vi "ExeCmd_async.vi"(4 "HighPrio":bool, 6 "CmdVIRef":refnum<vi>, 8 "ErrorIn":errorcluster, 9 "NameOfVi2Call(optional)":string, 10 "CmdData":variant, 11 "YActorIn":refnum<class "YActor.lvclass">) -> (0 "ErrorOut":errorcluster)   [LabVIEW 2021, in "YActor.lvclass"]
uses:
  YActor.lvclass
  YActor.lvclass/YActor.ctl
  private/CmdCtrl.ctl
  AsyncErrorHandling.ctl
  private/CallMode.ctl
  private/VINameProperty.vi
  InlineReferencePool.vi
panel:
  # "Do not use this VI in a loop where different Cmd VI references are routed.\nThis will cause the execution of the first called command VI only"
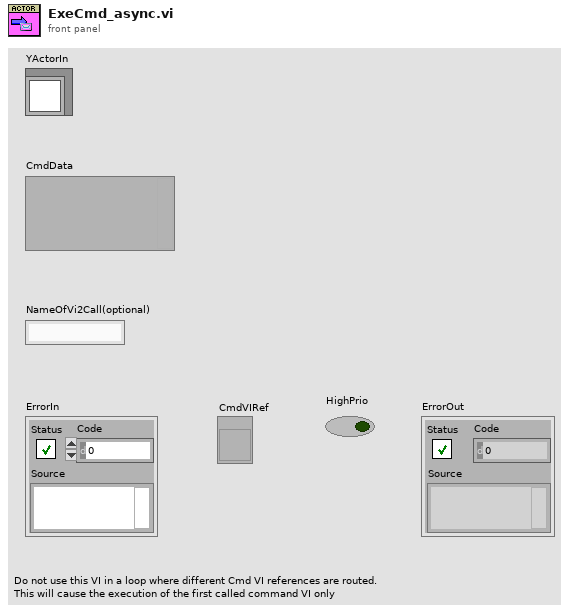
[diagram p1: front panel]
types:
  T1 = typedef "YActor.lvclass/CallMode.ctl" = enum16{"Standard", "Call&Collect"}
  T2 = typedef "YActor.lvclass/CmdCtrl.ctl" = cluster{"CmdData":variant, "CommandVI":string, "ReplyQ":i64, "Error":errorcluster, "Msg#":u32, "AsyncErrorHandling":T3, "CallMode":T1, "Source":string}
  T3 = typedef "YActor.lvclass/AsyncErrorHandling.ctl" = enum16{"Return after executing sync command", "Return before executing sync command", "Don't return error"}
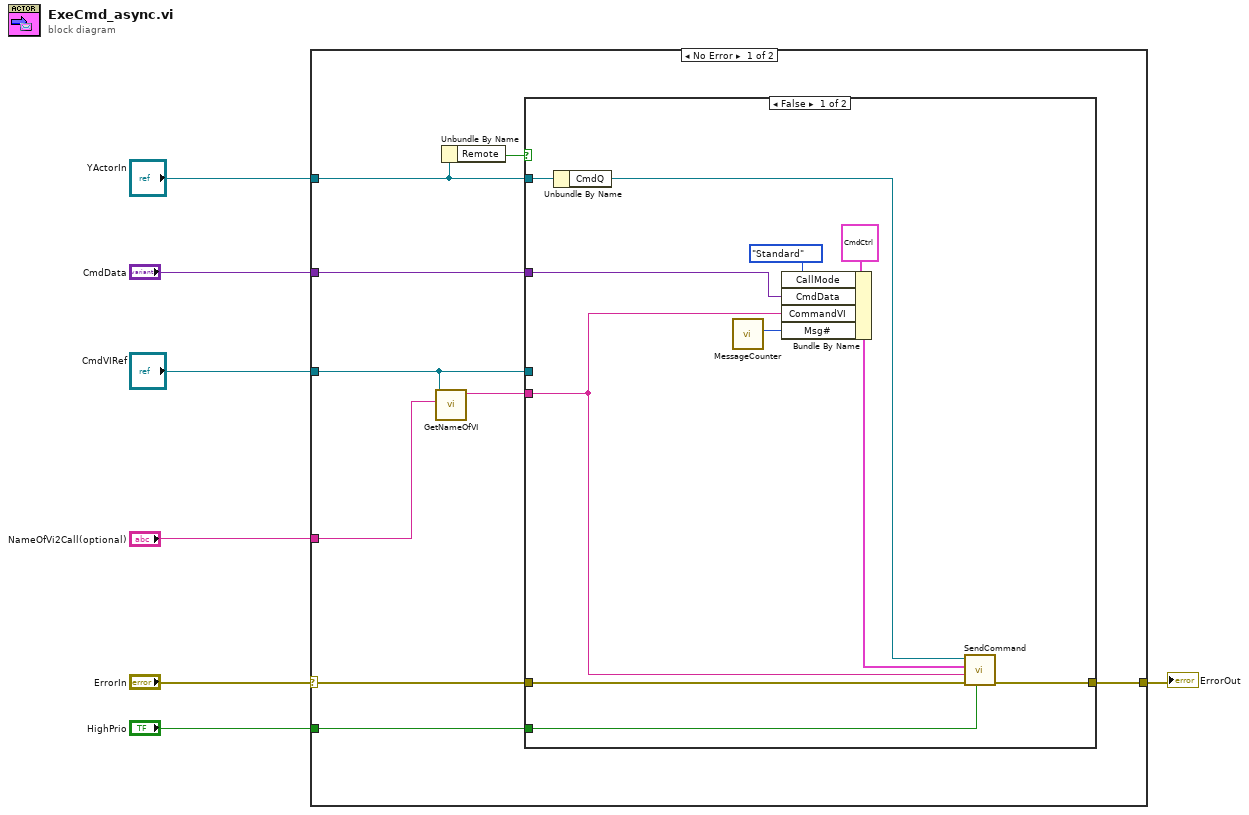
[diagram p0: block diagram]
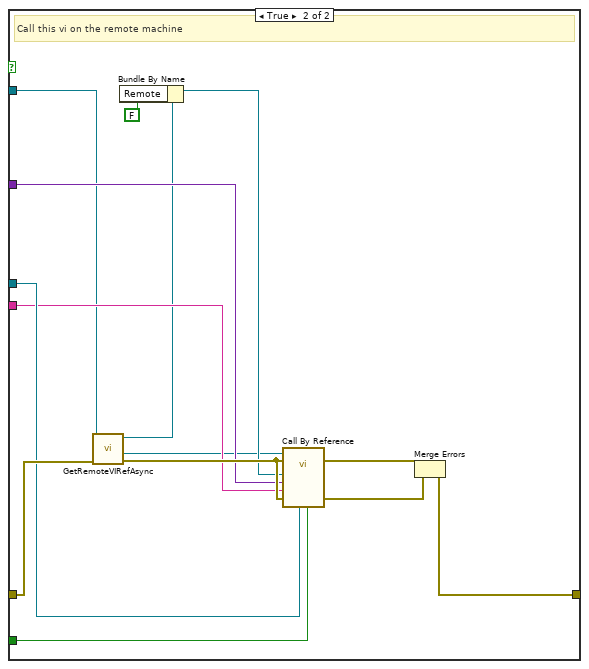
[diagram p2: hidden frame]
diagram:
  n1 = case shown="No Error" "ErrorIn" {
    selector: "ErrorIn" -> [w16 w42]
    tunnel: [w15 w42] -> w6
    tunnel: "YActorIn" -> [w12 _]
    tunnel: "CmdData" -> [w13 _]
    tunnel: "CmdVIRef" -> [w10 _]
    tunnel: "HighPrio" -> [w14 _]
    tunnel: "NameOfVi2Call(optional)" -> [w9 _]
    frame No Error {
      n2 = call "GetNameOfVI.vi"("NameOfVi2Call(optional)"=w9, "VIIn"=w10) -> ("Name"=w8:string)  [unwired: 9 in]
      n3 = Unbundle By Name(w12) -> ("Remote"=w11:bool)
      n4 = case shown="False" w11 {
        tunnel: w12 -> [w25 w30]
        tunnel: w16 -> [w27 w38]
        tunnel: w14 -> [w17 w32]
        tunnel: w13 -> [w22 w34]
        tunnel: w10 -> [_ w33]
        tunnel: [w26 w37] -> w15
        tunnel: w8 -> [w18 w31]
        frame False {
          n5 = Unbundle By Name(w25) -> ("CmdQ"=w20:refnum<queue>)
          n6 = call "MessageCounter.vi"() -> ("Msg#"=w23:u32)  [unwired: 11 in]
          n7 = Bundle By Name(cluster=T2 {"CmdData"=variant(refnum<class> refnum), "CommandVI"="", "ReplyQ"=0, "Error"={"Status"=FALSE, "Code"=0, "Source"=""}, "Msg#"=0, "AsyncErrorHandling"=enum."Return after executing sync command", "CallMode"=enum."Standard", "Source"=""} ("CmdCtrl"), "CallMode"=CallMode."Standard", "CmdData"=w22, "CommandVI"=w18, "Msg#"=w23) -> (w19:T2)
          n8 = call "SendCommand.vi"("HighPrio"=w17, "ErrorIn"=w27, "Name"=w18, "CmdCtrl"=w19, "QueueIn"=w20) -> ("ErrorOut"=w26:errorcluster)  [unwired: 6 in]
        }
        frame True {
          # "Call this vi on the remote machine"
          n9 = call "GetRemoteVIRefAsync.vi"("ErrorIn"=w38, "YActorIn"=w30) -> ("ErrorOut"=w41:errorcluster, "VIRef"=w28:refnum<vi>, "YActorOut"=w29:refnum<class "YActor.lvclass">)  [unwired: 7 in]
          n10 = Bundle By Name(cluster=w29, "Remote"=FALSE ("Remote.Remote?")) -> (w36:refnum<class "YActor.lvclass">)
          n11 = call-by-ref "?"(reference=w28, error in=w41, "High Prio"=w32, "Cmd VI ref"=w33, 8:"error in (no error)"=w41, "NameOfVi2Call (optional)"=w31, "Cmd Data"=w34, "reference in"=w36) -> (error out=w40:errorcluster, 0:"error out"=w39:errorcluster)  [unwired: 5 in, 1 out]
          n12 = Merge Errors(w40, w39) -> (w37:errorcluster)
        }
      }
    }
    frame Error {
    }
  }
  "ErrorOut" <- w6
